vi "Save_Text_Big_Array_to_Excel.vi"(8 "start Position":cluster{"row":i32, "column":i32}={"row"=2, "column"=0}, 9 "error in (no error)":errorcluster, 10 "report in":refnum<class "NI_report.lvclass">, 11 "배열":string[][](array[string])) -> (0 "Next position":cluster{"row":i32, "column":i32}, 1 "error out":errorcluster, 3 "report out":refnum<class "NI_report.lvclass">)   [LabVIEW 2015]
uses:
  <vilib>/Utility/NIReport.llb/NI_report.lvclass
  <vilib>/addons/_office/excel.llb/Excel Easy Table (str).vi
  <vilib>/addons/_office/NI_ReportGenerationToolkit.lvlib
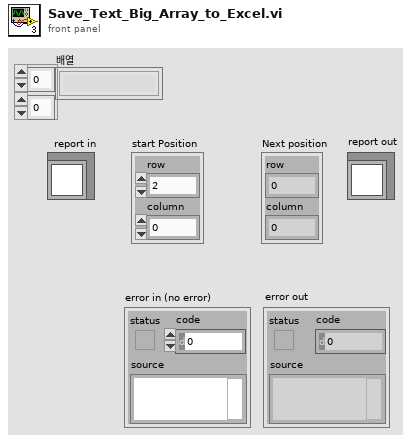
[diagram p1: front panel]
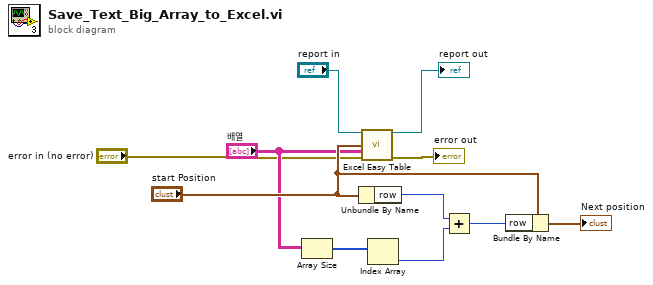
[diagram p0: block diagram]
diagram:
  n1 = Array Size(array="배열") -> (size(s)=w7:i32[])
  n2 = Unbundle By Name("start Position") -> ("row"=w8:i32)
  n3 = call-poly <vilib>:"Excel Easy Table.vi"("report in"="report in", "start (0, 0)"="start Position", "text data"="배열", "error in (no error)"="error in (no error)") -> ("report out"=→"report out":refnum<class "NI_report.lvclass">, "error out"=→"error out":errorcluster)  [unwired: 7 in, 3 out]
  n4 = Index Array(array=w7) -> (element=w9:i32)  [unwired: 1 in]
  n5 = Add(x=w8, y=w9) -> (x+y=w11:i32)
  n6 = Bundle By Name(cluster="start Position", "row"=w11) -> (→"Next position":cluster{"row":i32, "column":i32})
